vi "File Upload.vi"(0 "Sift Client in":refnum<class "Sift Client.lvclass">, 1 "Filepath":string, 2 "Entity ID":string, 3 "Entity Type":T1, 4 "Description":string, 5 "error in (no error)":errorcluster) -> (14 "Sift Client out":refnum<class "Sift Client.lvclass">, 19 "error out":errorcluster)   [LabVIEW 2024, in "Sift Client.lvlib" / "Sift Client.lvclass"]
doc: "Uploads an arbitrary file pointed to by Filepath and attaches it to the provided Entity ID."
uses:
  Sift Client.lvclass
  Private/Typedefs/Messages/File Attachment Upload Request.ctl
  Types/Entity Type.ctl
  Private/Typedefs/Messages/Video Metadata.ctl
  Private/Typedefs/Messages/Image Metadata.ctl
  Private/Typedefs/Messages/Metadata Type.ctl
  Private/Typedefs/Messages/JSON Request.ctl
  Sift Client.lvclass/Sift Client.ctl
  Sift Client.lvlib
  <vilib>/addons/_JKI.lib/Serialization/JSON/JKI JSON Serialization.lvlib
panel:
  in  "JSON Request":T2
  in  "File Attachment Upload Request":T3={"uri"="", "apikey"="", "filepath"="", "entity_id"="", "description"="", "entity_type"=enum."runs", "video_metadata"={"duration_seconds"=0.0, "timestamp"=timestamp(0 s since 1904-01-01), "height"=0, "width"=0}, "image_metadata"={"height"=0, "width"=0}, "metadata_type"=enum."image"}
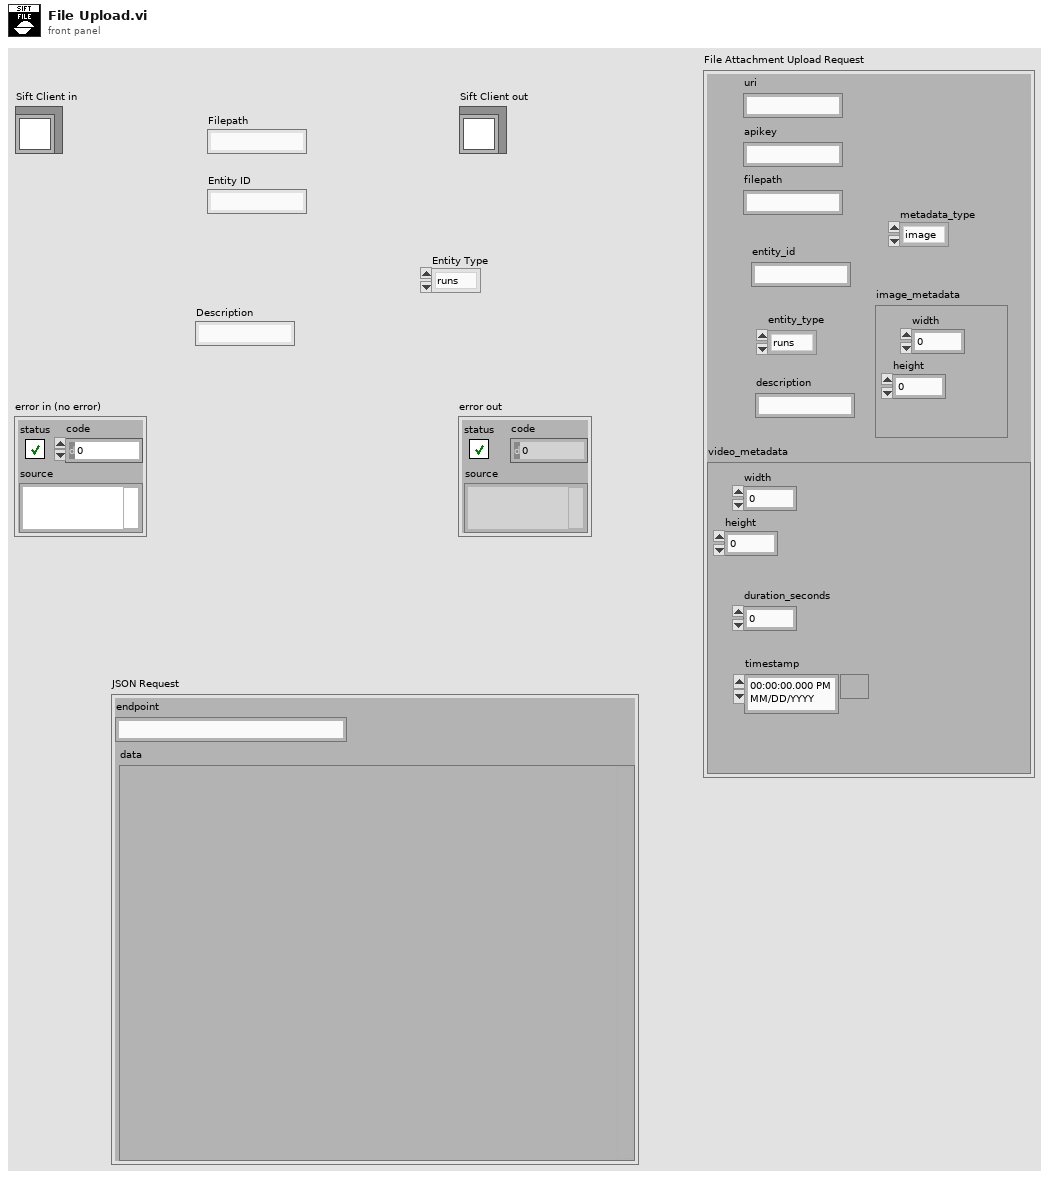
[diagram p1: front panel]
types:
  T1 = typedef "Sift Client.lvlib/Entity Type.ctl" = enum16{"runs", "annotations", "annotation_logs"}
  T2 = typedef "Sift Client.lvlib/JSON Request.ctl" = cluster{"endpoint":string, "data":variant}
  T3 = typedef "Sift Client.lvlib/File Attachment Upload Request.ctl" = cluster{"uri":string, "apikey":string, "filepath":string, "entity_id":string, "description":string, "entity_type":T1, "video_metadata":T4, "image_metadata":T5, "metadata_type":T6}
  T4 = typedef "Sift Client.lvlib/Video Metadata.ctl" = cluster{"duration_seconds":dbl, "timestamp":timestamp, "height":i32, "width":i32}
  T5 = typedef "Sift Client.lvlib/Image Metadata.ctl" = cluster{"height":i32, "width":i32}
  T6 = typedef "Sift Client.lvlib/Metadata Type.ctl" = enum16{"none", "image", "video"}
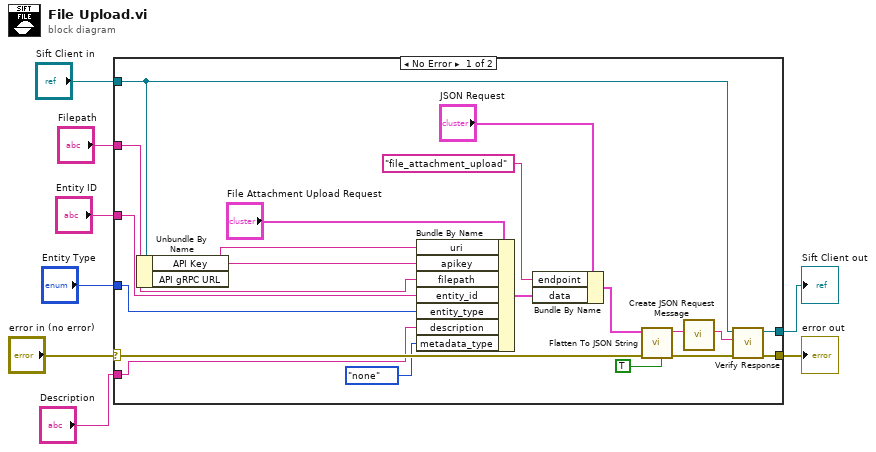
[diagram p0: block diagram]
diagram:
  n1 = case shown="No Error" "error in (no error)" {
    selector: "error in (no error)" -> [w20 w30]
    tunnel: [w19 w30] -> w7
    tunnel: [w18 w29] -> w5
    tunnel: "Sift Client in" -> [w11 w29]
    tunnel: "Entity Type" -> [w15 _]
    tunnel: "Entity ID" -> [w14 _]
    tunnel: "Filepath" -> [w13 _]
    tunnel: "Description" -> [w12 _]
    frame No Error {
      n2 = Unbundle By Name(w11) -> ("API Key"=w16:string, "API gRPC URL"=w17:string)
      n3 = Bundle By Name(cluster="File Attachment Upload Request", "uri"=w17, "apikey"=w16, "filepath"=w13, "entity_id"=w14, "entity_type"=w15, "description"=w12, "metadata_type"=Metadata_Type."none") -> (w26:T3)
      n4 = Bundle By Name(cluster="JSON Request", "endpoint"="file_attachment_upload", "data"=w26) -> (w21:T2)
      n5 = call <vilib>:"Flatten To JSON String.vi"("Enums As String (F)"=TRUE, "error in"=w20, "Variant"=w21) -> ("error out"=w22:errorcluster, "JSON String"=w24:string)  [unwired: 7 in]
      n6 = call "Create JSON Request Message.vi"("Data"=w24) -> ("Message"=w23:string)  [unwired: 10 in]
      n7 = call-dynamic "Verify Response.vi"("error in (no error)"=w22, "Message"=w23, "Sift Client in"=w11) -> ("error out"=w19:errorcluster, "Sift Client out"=w18:refnum<class "Sift Client.lvclass">)  [unwired: 6 in, 1 out]
    }
    frame Error {
    }
  }
  "error out" <- w7
  "Sift Client out" <- w5
